vi "STFT Spectrograms.vi"(6 "energy conservation?":bool=TRUE, 7 "time-freq config":T1={"force freq bins to power of 2?"=TRUE, "exclude Nyquist frequency?"=TRUE}, 8 "window parameter":dbl=nan, 9 "window info":cluster{"type":T2, "length":i32}={"type"=1, "length"=64} {"type" items=["Rectangle"=0, "Hanning"=1, "Hamming"=2, "Blackman-Harris"=3, "Exact Blackman"=4, "Blackman"=5, "Flat Top"=6, "4 Term B-Harris "=7, "7 Term B-Harris"=8, "Low Sidelobe"=9, "Blackman Nuttall"=11, "Triangle"=30, "Bartlett-Hanning"=31, "Bohman"=32, "Parzen"=33, "Welch"=34, "Kaiser"=60, "Dolph-Chebyshev"=61, "Gaussian"=62]}, 10 "time-freq sampling info":cluster{"time steps":i32, "frequency bins":i32}={"time steps"=-1, "frequency bins"=512}, 11 "X":dbl[](array[numeric])) -> (0 "error":i32, 3 "STFT Spectrogram {X}":dbl[][](array[numeric]))   [LabVIEW 2017, in "NI_Gmath.lvlib"]
doc: "Computes the signal energy distribution in the joint time-frequency domain, using the short-time Fourier transform (STFT) algorithm."
uses:
  NI_Gmath.lvlib
  windowTd.ctl
  Unit Vector (DBL).vi
  Real FFT.vi
  Scaled Time Domain Window (DBL).vi
  NI_AALBase.lvlib
  NI_AALPro.lvlib
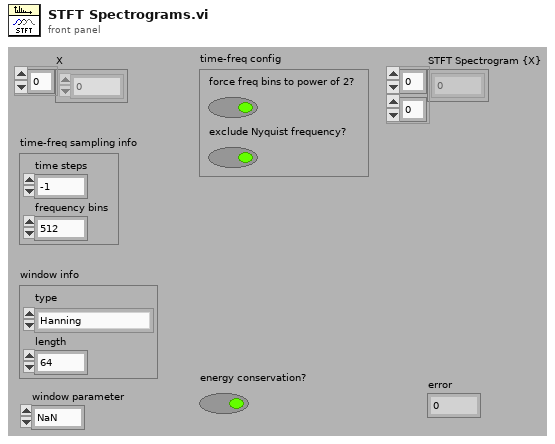
[diagram p1: front panel]
types:
  T1 = cluster{"force freq bins to power of 2?":bool, "exclude Nyquist frequency?":bool}
  T2 = typedef "NI_AALPro.lvlib/windowTd.ctl" = u32
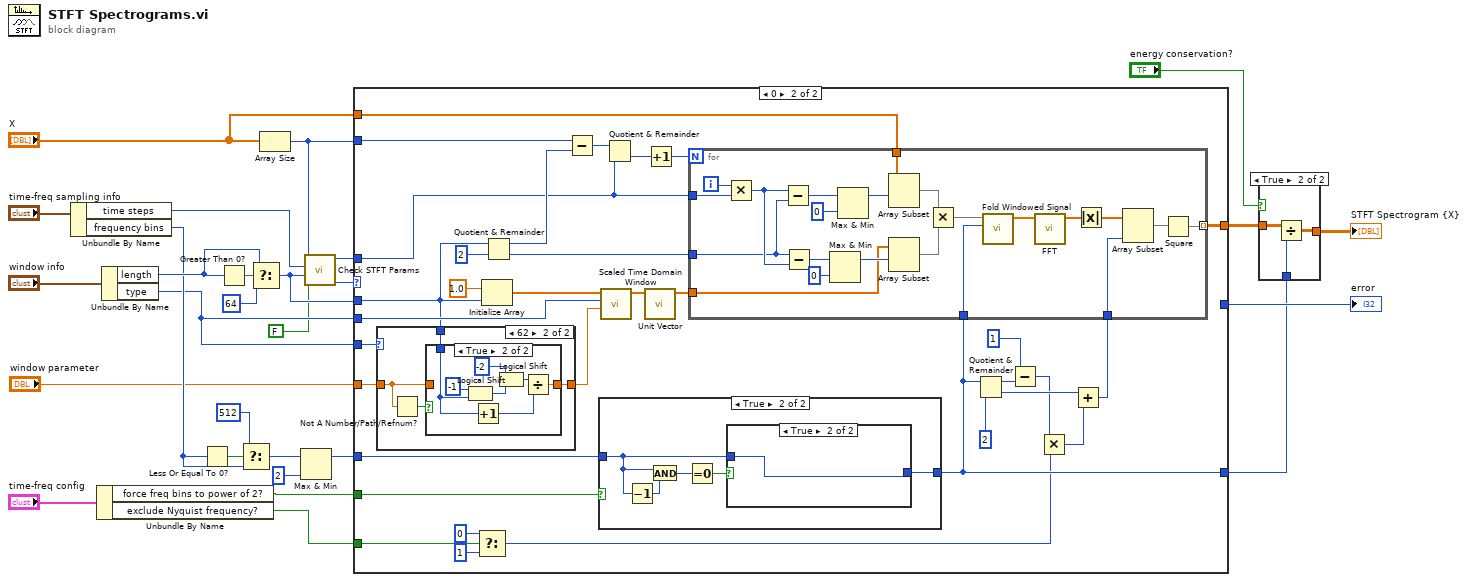
[diagram p0: block diagram]
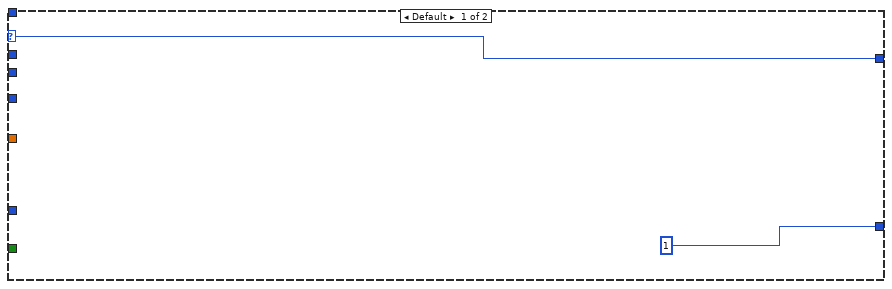
[diagram p3: hidden frame]
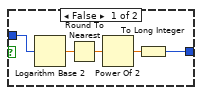
[diagram p7: hidden frame]
diagram:
  n1 = Unbundle By Name("time-freq sampling info") -> ("time steps"=w21:i32, "frequency bins"=w9:i32)
  n2 = Unbundle By Name("time-freq config") -> ("force freq bins to power of 2?"=w16:bool, "exclude Nyquist frequency?"=w15:bool)
  n3 = Unbundle By Name("window info") -> ("length"=w19:i32, "type"=w3:T2)
  n4 = Less Or Equal To 0?(x=w9) -> (x <= 0?=w10:bool)
  n5 = Greater Than 0?(x=w19) -> (x > 0?=w24:bool)
  n6 = Select(t=512, s=w10, f=w9) -> (s? t:f=w6:i32)
  n7 = Select(t=w19, s=w24, f=64) -> (s? t:f=w8:i32)
  n8 = Array Size(array="X") -> (size(s)=w27:i32)
  n9 = Max & Min(x=w6, y=2) -> (max(x,y)=w4:i32)  [unwired: 1 out]
  n10 = call "Check STFT Params.vi"("compare signal and window?"=FALSE, "windows length"=w8, "time increment"=w21, "len(X)"=w27) -> ("error"=w26:i32, "time step out"=w18:i32)  [unwired: 6 in]
  n11 = case shown="0" w26 {
    selector: w26 -> [w30 _]
    tunnel: w3 -> [_ w45]
    tunnel: "X" -> [_ w52]
    tunnel: [_ w46] -> w13
    tunnel: w27 -> [_ w58]
    tunnel: [w30 _] -> w25
    tunnel: w18 -> [_ w55]
    tunnel: w16 -> [_ w59]
    tunnel: w15 -> [_ w49]
    tunnel: [1 ("frequency bins") w39] -> w11
    tunnel: w8 -> [_ w44]
    tunnel: w4 -> [_ w43]
    tunnel: w3 -> [_ w41]
    tunnel: "window parameter" -> [_ w31]
    frame Default {
    }
    frame 0 {
      n12 = case shown="62" w41 {
        tunnel: w44 -> [_ w68]
        tunnel: [w64 w67] -> w42
        tunnel: w31 -> [w64 w65]
        frame 0, Default {
        }
        frame 62 {
          n13 = Not A Number/Path/Refnum?(number/path/refnum=w65) -> (NaN/Path/Refnum?=w66:bool)
          n14 = case shown="True" w66 {
            tunnel: w68 -> [_ w72]
            tunnel: [w69 w70] -> w67
            tunnel: w65 -> [w69 _]
            frame False {
            }
            frame True {
              n15 = Logical Shift(y=-1, x=w72) -> (x << y=w75:i32)
              n16 = Increment(x=w72) -> (x+1=w71:i32)
              n17 = Logical Shift(y=-2, x=w75) -> (x << y=w76:i32)
              n18 = Divide(x=w76, y=w71) -> (x/y=w70:dbl)
            }
          }
        }
      }
      n19 = Select(t=0, s=w49, f=1) -> (s? t:f=w37:i32)
      n20 = Initialize Array(1.0 ("element"), w44) -> (w61:dbl[])
      n21 = Quotient & Remainder(x=w44, y=2) -> (x-y*floor(x/y)=w57:i32, floor(x/y)=w50:i32)
      n22 = Subtract(x=w58, y=w57) -> (x-y=w56:i32)
      n23 = case shown="True" w59 {
        tunnel: w43 -> [w99 w101]
        tunnel: [w99 w100] -> w39
        frame False {
        }
        frame True {
          n24 = Decrement(x=w101) -> (x-1=w104:i32)
          n25 = And(x=w101, y=w104) -> (x .and. y?=w103:i32)
          n26 = Equal To 0?(x=w103) -> (x = 0?=w102:bool)
          n27 = case shown="True" w102 {
            tunnel: w101 -> [w109 w110]
            tunnel: [w105 w110] -> w100
            frame False {
              n28 = Logarithm Base 2(1:w109) -> (0:w108:dbl)
              n29 = Round To Nearest(number=w108) -> (nearest integer value=w107:dbl)
              n30 = Power Of 2(x=w107) -> (2^x=w106:dbl)
              n31 = To Long Integer(number=w106) -> (32bit integer=w105:i32)
            }
            frame True {
            }
          }
        }
      }
      n32 = call-poly "Scaled Time Domain Window.vi"("window parameter"=w42, "window"=w45, "X"=w61) -> ("Windowed X"=w60:dbl[])  [unwired: 6 in, 2 out]
      n33 = Quotient & Remainder(x=w56, y=w55) -> (floor(x/y)=w54:i32)  [unwired: 1 out]
      n34 = call-poly "Unit Vector.vi"("Input Vector"=w60) -> ("Unit Vector"=w51:dbl[])  [unwired: 8 in, 2 out]
      n35 = Increment(x=w54) -> (x+1=w53:i32)
      n36 = Quotient & Remainder(x=w39, y=2) -> (x-y*floor(x/y)=w34:i32, floor(x/y)=w35:i32)
      n37 = Subtract(x=1, y=w34) -> (x-y=w32:i32)
      n38 = Multiply(x=w32, y=w37) -> (x*y=w36:i32)
      n39 = Add(x=w35, y=w36) -> (x+y=w38:i32)
      n40 = for {
        N: w53 -> [_]
        tunnel: w50 -> [w84]
        tunnel: w52 -> [w98]
        tunnel: w55 -> [w79]
        tunnel: w51 -> [w94]
        tunnel: [w86] -> w46 mode=indexing
        tunnel: w39 -> [w78]
        tunnel: w38 -> [w77]
        i -> [w80]
        n41 = Multiply(x=w80, y=w79) -> (x*y=w85:i32)
        n42 = Subtract(x=w85, y=w84) -> (x-y=w81:i32)
        n43 = Subtract(x=w84, y=w85) -> (x-y=w97:i32)
        n44 = Max & Min(x=w97, y=0) -> (max(x,y)=w95:i32)  [unwired: 1 out]
        n45 = Max & Min(x=w81, y=0) -> (max(x,y)=w82:i32)  [unwired: 1 out]
        n46 = Array Subset(array=w98, index=w82) -> (w93:dbl[])  [unwired: 1 in]
        n47 = Array Subset(array=w94, index=w95) -> (w92:dbl[])  [unwired: 1 in]
        n48 = Multiply(x=w93, y=w92) -> (x*y=w91:dbl[])
        n49 = call "Fold Windowed Signal.vi"("frequency bins"=w78, "Windowed Signal"=w91) -> ("Folded Signal"=w90:dbl[])  [unwired: 9 in]
        n50 = call-poly "FFT.vi"("X"=w90) -> ("FFT {X}"=w89:cdb[])  [unwired: 9 in, 1 out]
        n51 = Absolute Value(x=w89) -> (abs(x)=w88:dbl[])
        n52 = Array Subset(array=w88, length=w77) -> (w87:dbl[])  [unwired: 1 in]
        n53 = Square(x=w87) -> (x^2=w86:dbl[])
      }
    }
  }
  "error" <- w25
  n54 = case shown="True" "energy conservation?" {
    tunnel: w13 -> [w111 w114]
    tunnel: w11 -> [_ w113]
    tunnel: [w111 w112] -> w12
    frame False {
    }
    frame True {
      n55 = Divide(x=w114, y=w113) -> (x/y=w112:dbl[][])
    }
  }
  "STFT Spectrogram {X}" <- w12
